vi "ni579x Construct Command Set LO Filter.vi"(0 "Register Bus":refnum<class "ni579x Register Bus v1 Host.lvclass">=refnum, 1 "scope":string, 5 "frequency [Hz]":dbl format="%#_6p", 11 "Error In":errorcluster) -> (4 "Register Bus (out)":refnum<class "ni579x Register Bus v1 Host.lvclass">, 6 "User Command":T1 {"User Command ID" items=["Set Clock Select"=0, "Set CLK OUT Source"=1, "DAC Sync User Start"=2, "DAC Sync User End"=3, "Enable Baseband Amp"=5, "Set Rx Attenuation Pre-LNA"=7, "Set Rx Attenuation Post-LNA"=8, "Set Tx Attenuation"=9, "Set LO Filter"=32, "Set Front End Filter"=33, "Enable LO"=34, "Set Routing Mux"=37, "Read Current Rev Lower"=240, "Read Current Rev Upper"=241, "Read Oldest Compat Rev Lower"=242, "Read Oldest Compat Rev Upper"=243, "Re-Initialize"=255]; "User Data 1" format="%x"; "User Data 0" format="%x"}, 15 "Error Out":errorcluster)   [LabVIEW 2013]
uses:
  <instrlib>/ni579x/Register Bus/v1/Host/ni579x Register Bus v1 Host.lvclass
  <instrlib>/ni579x/Config/v1/Shared/Types/ni579x User Command.ctl
  <instrlib>/ni579x/Config/v1/Shared/Types/ni579x User Command ID.ctl
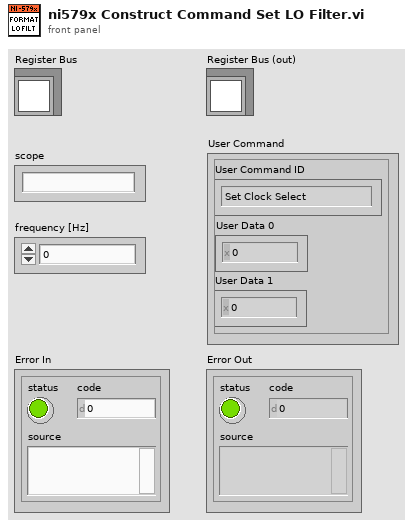
[diagram p1: front panel]
types:
  T1 = typedef "ni579x User Command.ctl" = cluster{"User Data 0":u8, "User Data 1":u8, "User Command ID":T2}
  T2 = typedef "ni579x User Command ID.ctl" = u8
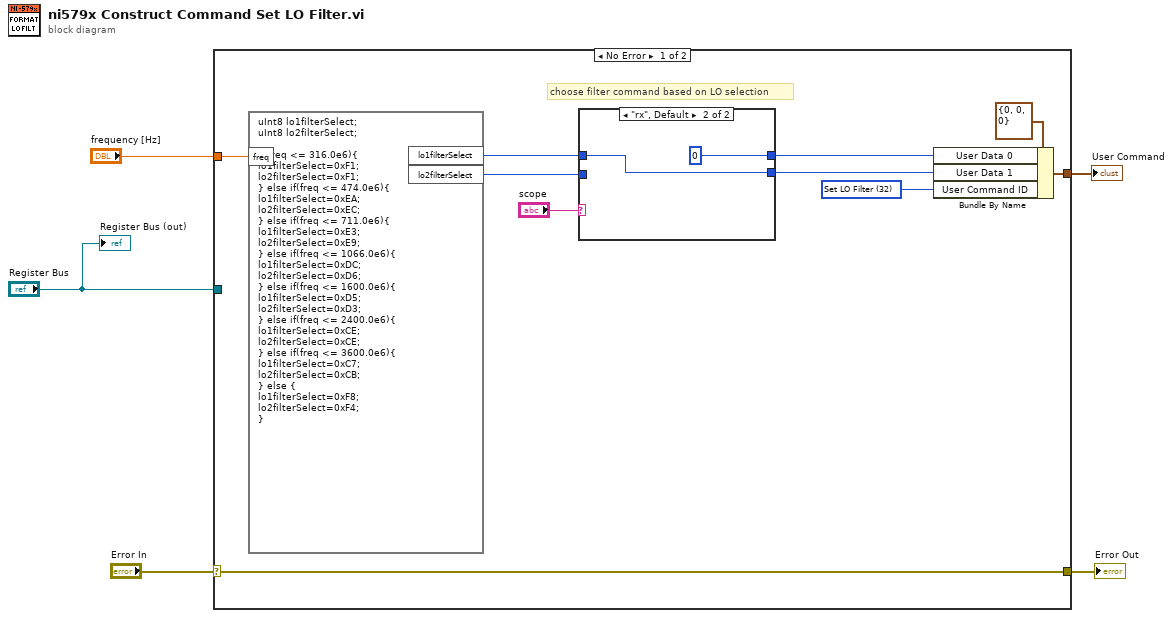
[diagram p0: block diagram]
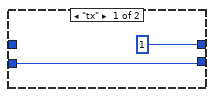
[diagram p2: hidden frame]
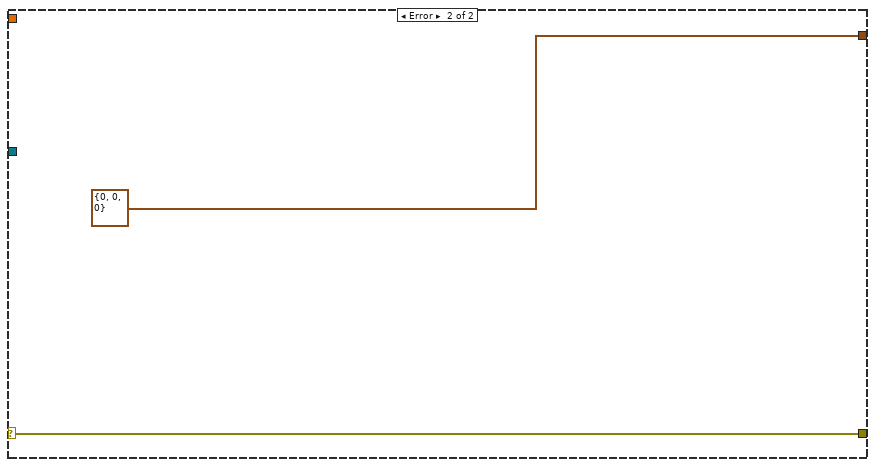
[diagram p3: hidden frame]
diagram:
  n1 = case shown="No Error" "Error In" {
    selector: "Error In" -> [w14 w21]
    tunnel: [w14 w21] -> w4
    tunnel: "Register Bus" -> [_ _]
    tunnel: "frequency [Hz]" -> [w13 _]
    tunnel: [w15 T1 {"User Data 0"=0, "User Data 1"=0, "User Command ID"=0} ("User Command")] -> w1
    frame No Error {
      w6 = T2 32 items=["Set Clock Select"=0, "Set CLK OUT Source"=1, "DAC Sync User Start"=2, "DAC Sync User End"=3, "Enable Baseband Amp"=5, "Set Rx Attenuation Pre-LNA"=7, "Set Rx Attenuation Post-LNA"=8, "Set Tx Attenuation"=9, "Set LO Filter"=32, "Set Front End Filter"=33, "Enable LO"=34, "Set Routing Mux"=37, "Read Current Rev Lower"=240, "Read Current Rev Upper"=241, "Read Oldest Compat Rev Lower"=242, "Read Oldest Compat Rev Upper"=243, "Re-Initialize"=255] ("User Command ID")
      # "choose filter command based on LO selection"
      n2 = formula code="uInt8 lo1filterSelect;\nuInt8 lo2filterSelect;\n\nif(freq <= 316.0e6){\nlo1filterSelect=0xF1;\nlo2filterSelect=0xF1;\n} else if(freq <= 474.0e6){\nlo1filterSelect=0xEA;\nlo2filterSelect=0xEC;\n} else if(freq <= 711.0e6){\nlo1filterSelect=0xE3;\nlo2filterSelect=0xE9;\n} else if(freq <= 1066.0e6){\nlo1filterSelect=0xDC;\nlo2filterSelect=0xD6;\n} else if(freq <= 1600.0e6){\nlo1filterSelect=0xD5;\nlo2filterSelect=0xD3;\n} else if(freq <= 2400.0e6){\nlo1filterSelect=0xCE;\nlo2filterSelect=0xCE;\n} else if(freq <= 3600.0e6){\nlo1filterSelect=0xC7;\nlo2filterSelect=0xCB;\n} else {\nlo1filterSelect=0xF8;\nlo2filterSelect=0xF4;\n}"("freq"=w13) -> ("lo1filterSelect"=w9:u8, "lo2filterSelect"=w8:u8)
      n3 = case shown="\"rx\", Default" "scope" {
        tunnel: [u8 1 u8 0] -> w10
        tunnel: w9 -> [_ w18]
        tunnel: w8 -> [w16 _]
        tunnel: [w16 w18] -> w7
        frame "tx" {
        }
        frame "rx", Default {
        }
      }
      n4 = Bundle By Name(cluster=T1 {"User Data 0"=0, "User Data 1"=0, "User Command ID"=0} ("User Command"), "User Data 0"=w10, "User Data 1"=w7, "User Command ID"=w6) -> (w15:T1)
    }
    frame Error {
    }
  }
  "Error Out" <- w4
  "User Command" <- w1
  "Register Bus (out)" <- "Register Bus"
